vi "PCS-Menu.vi"() -> ()   [LabVIEW 2011]
panel:
  in  "PIT Button 3":bool
  in  "Auto Button 2":bool
  in  "Manual Button":bool
  in  "stop":bool
  # "PCS - Pressure cycling system"
  # "PCS - Pressure cycling system"
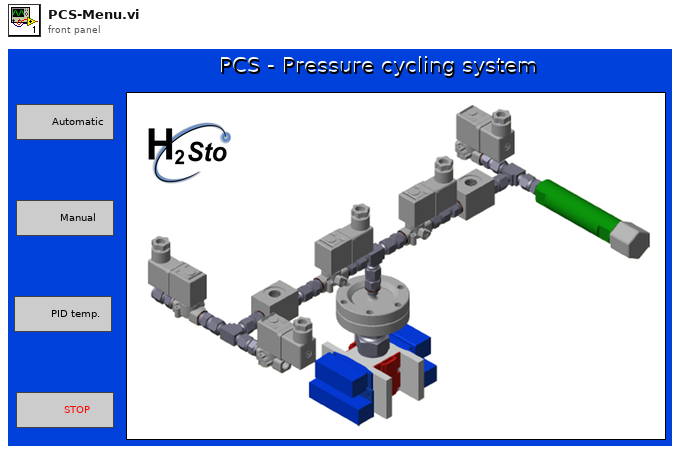
[diagram p1: front panel]
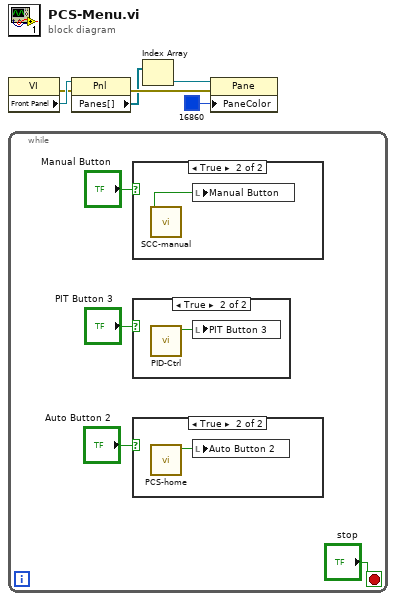
[diagram p0: block diagram]
diagram:
  n1 = property class="VI"() -> (error out=w2:errorcluster, "Front Panel"=w3:refnum<vi>)  [unwired: 2 in, 1 out]
  n2 = while {
    stop <- "stop" stop-if-true
    n3 = case shown="True" "Manual Button" {
      frame False {
      }
      frame True {
        n4 = call "SCC-manual.vi"() -> ("Boolean"=w11:bool)  [unwired: 11 out]
        n5 = local write "Manual Button"(w11) -> ()
      }
    }
    n6 = case shown="True" "PIT Button 3" {
      frame False {
      }
      frame True {
        n7 = call "PID-Ctrl.vi"() -> (".not. x?"=w12:bool)  [unwired: 11 in]
        n8 = local write "PIT Button 3"(w12) -> ()
      }
    }
    n9 = case shown="True" "Auto Button 2" {
      frame False {
      }
      frame True {
        n10 = call "PCS-home.vi"() -> ("Stop"=w13:bool)  [unwired: 11 in]
        n11 = local write "Auto Button 2"(w13) -> ()
      }
    }
  }
  n12 = property class="Pnl"(reference=w3, error in=w2) -> (error out=w6:errorcluster, "Panes[]"=w4:refnum<vi>[])  [unwired: 1 out]
  n13 = Index Array(array=w4) -> (element=w5:refnum<vi>)  [unwired: 1 in]
  n14 = property class="Pane"(reference=w5, error in=w6, "PaneColor"=u32 16860 ("Color Box")) -> ()  [unwired: 2 out]
